vi "OFDM-SIM硬件.vi"() -> ()   [LabVIEW 2018]
uses:
  <instrlib>/niUSRP/niUSRP Write Tx Data (CDB Cluster).vi
panel:
  in  "error in (no error)":errorcluster
  in  "?":enum32{"硬件参数", "调制参数"}(tab)
  in  "硬件参数":T1={"IP地址"="192.168.10.2", "IQ采样率(samples/s)"=500000.0, "载波频率(Hz)"=915000000.0, "增益(dB)"=20.0, "有效天线"="TX1", "信道列表(channel list)"="0"} {"增益(dB)" format="%#_6f"; "载波频率(Hz)" format="%#_6p"; "IQ采样率(samples/s)" format="%#_6p"}
  in  "调制参数 in":T2={"TX 过采样因子"=8.0, "脉冲成形参数"={"调制类型"=enum."PSK", "脉冲成形滤波器"=enum."Raised Cosine", "滤波器参数"=0.5, "滤波长度 (码元)"=8}} {"脉冲成形参数"."滤波器参数" format="%.2f"}
  out "coerced gain":dbl format="%#_6f"
  out "coerced carrier frequency":dbl=100000.0 format="%#_6p"
  out "coerced IQ rate":dbl=100000.0 format="%#_6p"
  out "error out":errorcluster
  in  "停止":bool
  out "Frame Length [samples]":i32
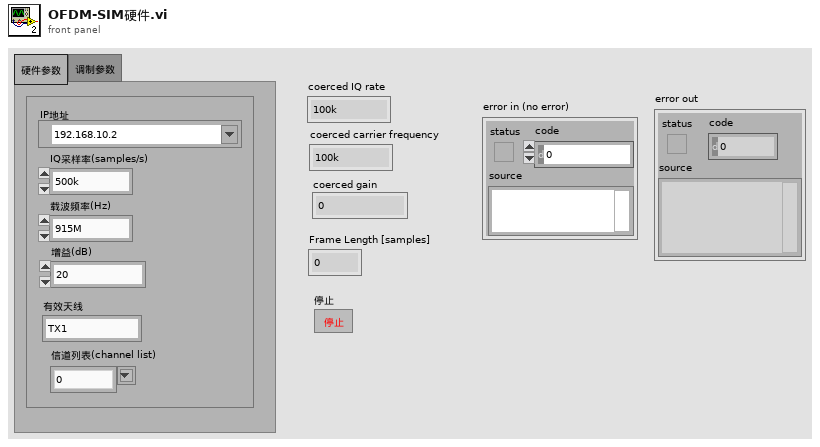
[diagram p1: front panel]
types:
  T1 = cluster{"IP地址":refnum<k15>, "IQ采样率(samples/s)":dbl, "载波频率(Hz)":dbl, "增益(dB)":dbl, "有效天线":string, "信道列表(channel list)":string}
  T2 = cluster{"TX 过采样因子":dbl, "脉冲成形参数":cluster{"调制类型":enum16{"FSK", "PSK", "QAM", "MSK", "PAM", "ASK", "CPM"}, "脉冲成形滤波器":enum16{"none", "Raised Cosine", "Root Raised Cos", "Gaussian"}, "滤波器参数":dbl, "滤波长度 (码元)":i32}}
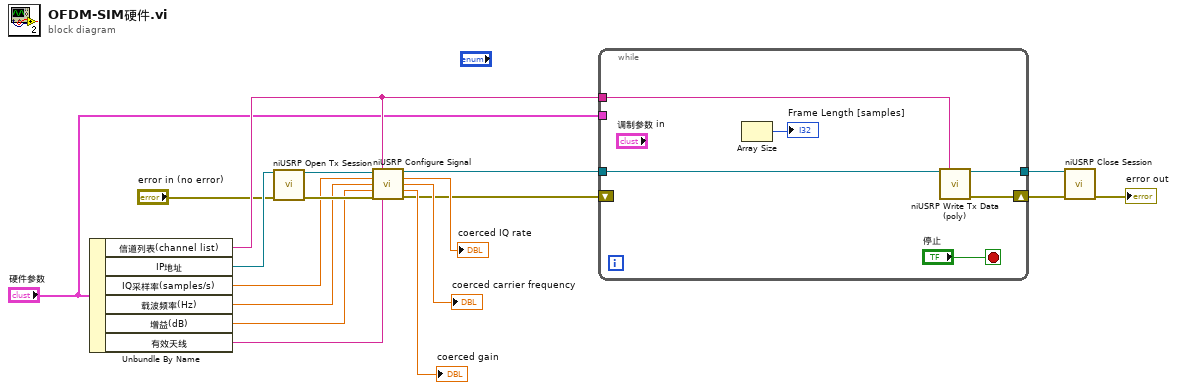
[diagram p0: block diagram]
diagram:
  n1 = Unbundle By Name("硬件参数") -> ("信道列表(channel list)"=w7:string, "IP地址"=w8:refnum<k15>, "IQ采样率(samples/s)"=w6:dbl, "载波频率(Hz)"=w5:dbl, "增益(dB)"=w4:dbl, "有效天线"=w3:string)
  n2 = call <instrlib>:"niUSRP Open Tx Session.vi"("device names"=w8, "error in (no error)"="error in (no error)") -> ("session handle out"=w17:refnum<k15>, "error out"=w18:errorcluster)  [unwired: 12 in]
  n3 = call <instrlib>:"niUSRP Configure Signal.vi"("session handle"=w17, "channel list"=w7, "IQ rate"=w6, "carrier frequency"=w5, "gain"=w4, "error in (no error)"=w18, "active antenna"=w3) -> ("session handle out"=w10:refnum<k15>, "coerced IQ rate"=→"coerced IQ rate":dbl, "coerced carrier frequency"=→"coerced carrier frequency":dbl, "coerced gain"=→"coerced gain":dbl, "error out"=w9:errorcluster)  [unwired: 4 in]
  n4 = while {
    tunnel: w10 -> [w29]
    tunnel: [w30] -> w16
    tunnel: w7 -> [w28]
    shift-right: [w27] -> w11
    shift-left: w9 -> [w24]
    tunnel: "硬件参数" -> [w23]
    stop <- "停止" stop-if-true
    n5 = Array Size() -> (array=w25:dbl[], size(s)=→"Frame Length [samples]":i32)
    n6 = call-poly <instrlib>:"niUSRP Write Tx Data (poly).vi"("session handle"=w29, "channel list"=w28) -> ("session handle out"=w30:refnum<k15>, "data"=w22:cluster{"t0":dbl, "dt":dbl, "Y":cdb[]}, "error in (no error)"=w20:errorcluster, "error out"=w27:errorcluster)  [unwired: 10 in]
  }
  n7 = call <instrlib>:"niUSRP Close Session.vi"("session handle"=w16, "error in (no error)"=w11) -> ("error out"=→"error out":errorcluster)  [unwired: 13 in]
